vi "publishRecommendedSettings.vi"(8 "error in (no error)":errorcluster, 11 "Model in":refnum<class "Model.lvclass">) -> (0 "error out":errorcluster, 3 "Model out":refnum<class "Model.lvclass">)   [LabVIEW 2016, in "Model.lvclass"]
doc: "Publish recommended settings through SAL. Is a string with comma separated value format."
uses:
  Model.lvclass
  ComponentTemplateCore/ComponentModel/ComponentModel/ConfigurationFileReader/ConfigurationFileReader.lvclass
  Typedefs/PubDataSV.ctl
  Typedefs/EXATypedefs.lvlib
  ts_sallv_exa/DataTypes/logevent_SettingVersions.ctl
  ts_sallv_exa/SALLV_EXA.lvlib
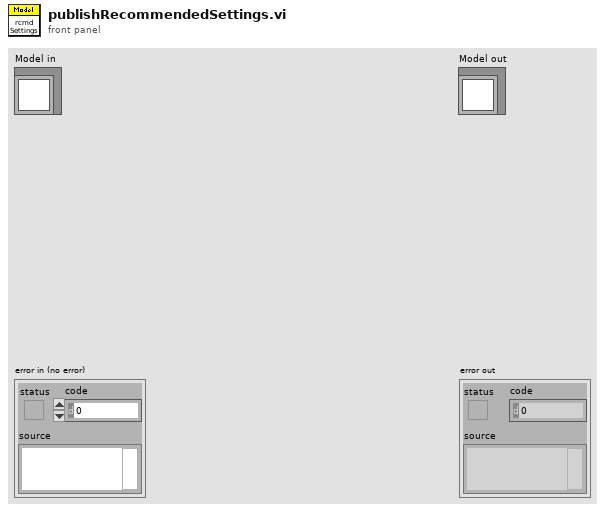
[diagram p1: front panel]
types:
  T1 = typedef "SALLV_EXA.lvlib/logevent_SettingVersions.ctl" = cluster{"recommendedSettingsLabels":string, "recommendedSettingsVersion":string, "priority":i32}
  T2 = typedef "EXATypedefs.lvlib/PubDataSV.ctl" = enum16{"DetailedState", "ErrorCode", "Heartbeat", "LoopTime_ms", "LoopTimeOutOfRange", "RejectedCommand", "SummaryState", "Timestamp", "SettingVersions", "SettingsApplied", "AppliedSettingsMatchStart"}
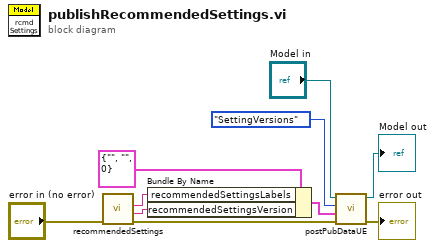
[diagram p0: block diagram]
diagram:
  n1 = call "recommendedSettings.vi"("error in (no error)"="error in (no error)") -> ("error out"=w6:errorcluster, "RecommendedSettingsLabels"=w1:string, "RecommendedSettingsVersions"=w4:string)  [unwired: 7 in, 1 out]
  n2 = Bundle By Name(cluster=T1 {"recommendedSettingsLabels"="", "recommendedSettingsVersion"="", "priority"=0} ("event data"), "recommendedSettingsLabels"=w4, "recommendedSettingsVersion"=w1) -> (w3:T1)
  n3 = call "postPubDataUE.vi"("error in (no error)"=w6, "value"=w3, "pubDataSV"=PubDataSV."SettingVersions", "Model in"="Model in") -> ("error out"=→"error out":errorcluster, "Model out"=→"Model out":refnum<class "Model.lvclass">)  [unwired: 6 in]
